vi "Start SPI Transaction.vi"(8 "error in":errorcluster, 9 "Start? (T)":bool=TRUE, 11 "SPI Engine Resources":T1={"To SPI Engine Data FIFO"="DLU To SPI Engine Data", "From SPI Engine Data FIFO"="SPI Engine to DLU Data", "Data to SPI Engine (Cache) Register"="Data to SPI Engine (Cache)", "SPI Settings to SPI Engine (Cache) Register"="SPI PHY Settings to SPI Engine (Cache)"}) -> (0 "error out":errorcluster, 1 "SPI Transaction Accepted?":bool, 3 "SPI Engine Resources":T1={"To SPI Engine Data FIFO"="DLU To SPI Engine Data", "From SPI Engine Data FIFO"="SPI Engine to DLU Data", "Data to SPI Engine (Cache) Register"="Data to SPI Engine (Cache)", "SPI Settings to SPI Engine (Cache) Register"="SPI PHY Settings to SPI Engine (Cache)"})   [LabVIEW 2015]
doc: "This VI sends \"Start Command\" to SPI Engine so that SPI Engine start bit-toggling on the DIO lines.\n\nNote: It is recommended to poll \"SPI Started?\" to ensure that the SPI transaction is started by SPI Engine"
uses:
  Controls/SPI Engine Resources.ctl
  <vilib>/rvi/DataTransferAndStorage/Container/Common/niFpgaContainerExecOnDevCompGetState.vi
  <vilib>/rvi/Emulation/niFpgaEmulationIsFPGAContextNoSignature.vi
  <vilib>/rvi/DataTransferAndStorage/Container/Common/niFpgaContainerGetUniqueNameForEmu.vi
  <vilib>/rvi/Memory/Memory_Emulation/niFpgaMemoryEmulationCacheClearOnFirstRun.vi
  <vilib>/rvi/Memory/Memory_Emulation/nirvimemoryEmulationManagerCache_MakeExclusive.vi
  <vilib>/rvi/Memory/Memory_Emulation/niFpgaMemoryEmulationValidateCache.vi
  <vilib>/rvi/Memory/Memory_Emulation/nirvimemoryEmulationManagerCache_InsertValue.vi
  <vilib>/Utility/error.llb/Clear Errors.vi
  <vilib>/rvi/Memory/Memory_Emulation/nirvimemoryEmulationManagerCache_ReleaseExclusive.vi
  <vilib>/rvi/Memory/Memory_Emulation/nirvimemoryEmulationManagerCache_GetValue.vi
  <vilib>/rvi/Memory/Memory_Emulation/nirvimemoryEmulationManagerCache_SetValue.vi
  <vilib>/rvi/Emulation/niFpgaProcessEmulError.vi
  <vilib>/rvi/Emulation/niFpgaSctlEmulationGetInTimedLoop.vi
  <vilib>/rvi/errors/niFpgaSetErrorForExecOnDevCompSimple.vi
  <vilib>/rvi/eio/common/nirviEmuReportErrorAndStop.vi
  <vilib>/rvi/FIFO/Fifo_Resource/nirvififoEmulationSetSize.vi
  <vilib>/rvi/FIFO/Fifo_Resource/nirviFifoEmulationQueueMgr.vi
  <instcachedir>/0/nirviFifoEmulationQueueMgr_E5CAEC123FF24DC58D834DCA3CDAA9B5.lvgen/nirviFifoEmulationQueueMgr_E5CAEC123FF24DC58D834DCA3CDAA9B5_006.vi
  <vilib>/rvi/FIFO/Fifo_Resource/nirvififoEmulationDetermineInputValidOut.vi
  <vilib>/rvi/FIFO/Fifo_Resource/nirvififoEmulationCreateLock.vi
  <vilib>/rvi/FIFO/Fifo_Resource/nirvififoEmulationObtainLock.vi
  <vilib>/rvi/FIFO/Fifo_Resource/nirvififoEmulationReleaseLock.vi
  <vilib>/rvi/occurrence/nirviWaitOnOccurrenceBase.vi
  <vilib>/rvi/errors/nirviReportUnexpectedCaseInternalError.vi
  <vilib>/rvi/errors/nirviReportUnexpectedCaseInternalError (U32).vi
  <vilib>/rvi/interface/RandomDataEmulation/niFpgaRandomDataHandleErrors.vi
  <vilib>/rvi/DataTransferAndStorage/Container/XNode/niFpgaContainer.xnode
  <vilib>/rvi/DataTransferAndStorage/Register/Emulation/niFpgaRegisterEmulationRefIn.vi
  <vilib>/rvi/FIFO/Fifo_Resource/niFpgaFifoEmulationRefIn.vi
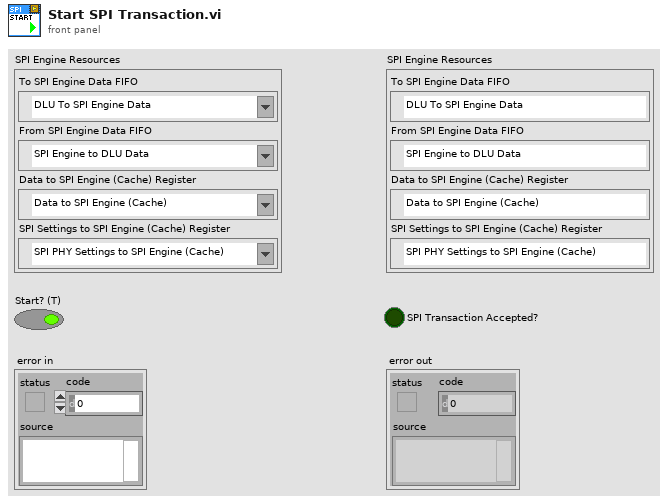
[diagram p1: front panel]
types:
  T1 = typedef "SPI Engine Resources.ctl" = cluster{"To SPI Engine Data FIFO":refnum<k21>, "From SPI Engine Data FIFO":refnum<k21>, "Data to SPI Engine (Cache) Register":refnum<k21>, "SPI Settings to SPI Engine (Cache) Register":refnum<k21>}
  T2 = cluster{"Chip Select ID":u8, "SPI Data":u64, "SPI PHY Settings":cluster{"Divide Value":u8, "Transfer Length (bits)":u8, "CS Asserted Polarity":bool, "Clock Polarity (CPOL)":bool, "Clock Phase (CPHA)":bool, "Lengthen MISO Setup":bool, "Direction Change Bit":u8, "MOSI Starts as Output":bool, "Tristatable MOSI":bool}}
  T3 = cluster{"Chip Select ID":u8, "SPI PHY Settings":cluster{"Divide Value":u8, "Transfer Length (bits)":u8, "CS Asserted Polarity":bool, "Clock Polarity (CPOL)":bool, "Clock Phase (CPHA)":bool, "Lengthen MISO Setup":bool, "Direction Change Bit":u8, "MOSI Starts as Output":bool, "Tristatable MOSI":bool}}
  T4 = cluster{"Divide Value":u8, "Transfer Length (bits)":u8, "CS Asserted Polarity":bool, "Clock Polarity (CPOL)":bool, "Clock Phase (CPHA)":bool, "Lengthen MISO Setup":bool, "Direction Change Bit":u8, "MOSI Starts as Output":bool, "Tristatable MOSI":bool}
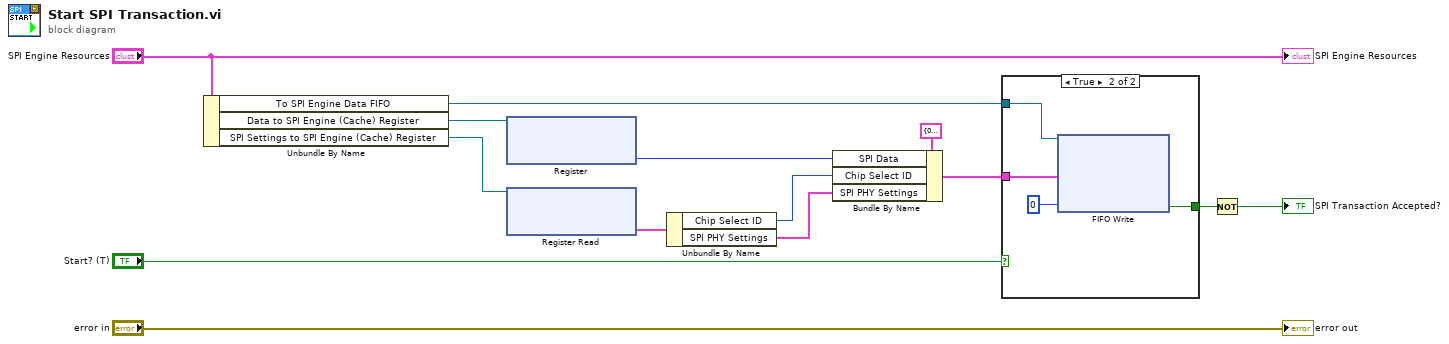
[diagram p0: block diagram]
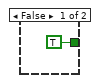
[diagram p2: hidden frame]
diagram:
  n1 = Unbundle By Name("SPI Engine Resources") -> ("To SPI Engine Data FIFO"=w12:refnum<k21>, "Data to SPI Engine (Cache) Register"=w10:refnum<k21>, "SPI Settings to SPI Engine (Cache) Register"=w9:refnum<k21>)
  n2 = xnode "Register"("Register In"=w10) -> ("Data"=w7:u64)  [unwired: 1 out]
  n3 = xnode "Register Read"("Register In"=w9) -> ("Data"=w6:T3)  [unwired: 1 out]
  n4 = Unbundle By Name(w6) -> ("Chip Select ID"=w5:u8, "SPI PHY Settings"=w4:T4)
  n5 = Bundle By Name(cluster=T2 {"Chip Select ID"=0, "SPI Data"=0, "SPI PHY Settings"={"Divide Value"=0, "Transfer Length (bits)"=0, "CS Asserted Polarity"=FALSE, "Clock Polarity (CPOL)"=FALSE, "Clock Phase (CPHA)"=FALSE, "Lengthen MISO Setup"=FALSE, "Direction Change Bit"=0, "MOSI Starts as Output"=FALSE, "Tristatable MOSI"=FALSE}} ("Element"), "SPI Data"=w7, "Chip Select ID"=w5, "SPI PHY Settings"=w4) -> (w2:T2)
  n6 = case shown="True" "Start? (T)" {
    tunnel: w12 -> [_ w19]
    tunnel: [TRUE ("Timed Out?") w18] -> w11
    tunnel: w2 -> [_ w16]
    frame False {
    }
    frame True {
      n7 = xnode "FIFO Write"("Element"=w16, "Timeout"=0, "FIFO In"=w19) -> ("Timed Out?"=w18:bool)  [unwired: 1 out]
    }
  }
  n8 = Not(x=w11) -> (.not. x?=→"SPI Transaction Accepted?":bool)
  "error out" <- "error in"
  "SPI Engine Resources" <- "SPI Engine Resources"
